vi "Drive Setting Modifier.vi"(0 "DT Input Modifier":T1, 1 "Creep Rate":dbl, 5 "Y Power Multiplier":dbl, 9 "Turn Power Multiplier":dbl, 11 "Axes[0]":dbl, 12 "Button[2]":bool, 13 "Axes[2]":dbl) -> (4 "Y Out":dbl, 6 "X Out":dbl)   [LabVIEW 2017]
uses:
  Common Code/DT Input Modifier.ctl
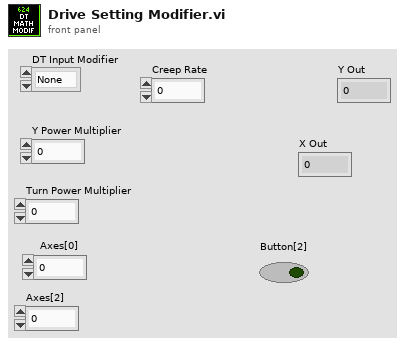
[diagram p1: front panel]
types:
  T1 = typedef "DT Input Modifier.ctl" = enum16{"None", "Square", "Cube"}
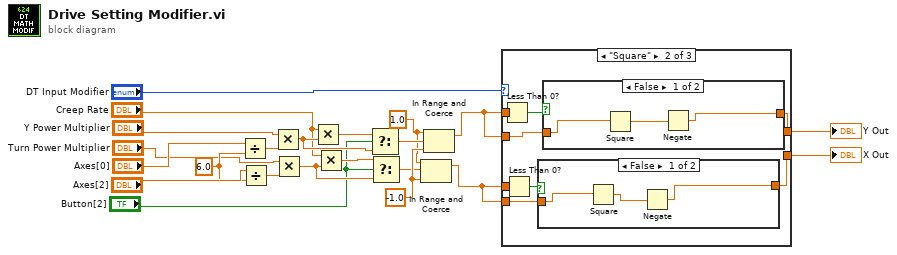
[diagram p0: block diagram]
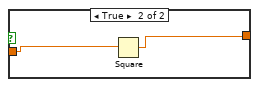
[diagram p3: hidden frame]
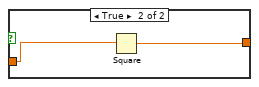
[diagram p4: hidden frame]
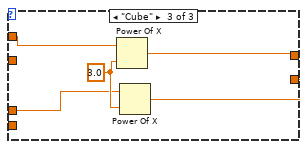
[diagram p5: hidden frame]
diagram:
  w7 = -1.0
  w6 = 1.0
  w19 = 6.0
  n1 = Divide(x="Axes[0]", y=w19) -> (x/y=w18:dbl)
  n2 = Divide(x="Axes[2]", y=w19) -> (x/y=w15:dbl)
  n3 = Multiply(x="Y Power Multiplier", y=w18) -> (x*y=w11:dbl)
  n4 = Multiply(x="Turn Power Multiplier", y=w15) -> (x*y=w14:dbl)
  n5 = Multiply(x="Creep Rate", y=w11) -> (x*y=w12:dbl)
  n6 = Multiply(x="Creep Rate", y=w14) -> (x*y=w13:dbl)
  n7 = Select(t=w12, s="Button[2]", f=w11) -> (s? t:f=w8:dbl)
  n8 = Select(t=w13, s="Button[2]", f=w14) -> (s? t:f=w5:dbl)
  n9 = In Range and Coerce(upper limit=w6, x=w5, lower limit=w7) -> (coerced(x)=w3:dbl)  [unwired: 1 out]
  n10 = In Range and Coerce(upper limit=w6, x=w8, lower limit=w7) -> (coerced(x)=w4:dbl)  [unwired: 1 out]
  n11 = case shown="\"Square\"" "DT Input Modifier" {
    tunnel: w3 -> [w24 w30 w46]
    tunnel: w4 -> [w23 w29 w45]
    tunnel: w4 -> [_ w28 _]
    tunnel: w3 -> [_ w27 _]
    tunnel: [w23 w26 w44] -> w2
    tunnel: [w24 w25 w43] -> w1
    frame "None", Default {
    }
    frame "Square" {
      n12 = Less Than 0?(x=w29) -> (x < 0?=w32:bool)
      n13 = Less Than 0?(x=w30) -> (x < 0?=w31:bool)
      n14 = case shown="False" w31 {
        tunnel: w27 -> [w34 w37]
        tunnel: [w33 w36] -> w25
        frame False {
          n15 = Square(x=w34) -> (x^2=w35:dbl)
          n16 = Negate(x=w35) -> (-x=w33:dbl)
        }
        frame True {
          n17 = Square(x=w37) -> (x^2=w36:dbl)
        }
      }
      n18 = case shown="False" w32 {
        tunnel: w28 -> [w40 w42]
        tunnel: [w38 w41] -> w26
        frame False {
          n19 = Square(x=w40) -> (x^2=w39:dbl)
          n20 = Negate(x=w39) -> (-x=w38:dbl)
        }
        frame True {
          n21 = Square(x=w42) -> (x^2=w41:dbl)
        }
      }
    }
    frame "Cube" {
      w47 = 3.0
      n22 = Power Of X(1:w47, 2:w45) -> (0:w44:dbl)
      n23 = Power Of X(1:w47, 2:w46) -> (0:w43:dbl)
    }
  }
  "Y Out" <- w2
  "X Out" <- w1
